vi "Get Boolean.vi"(1 "Name":string) -> (0 "Value":bool)   [LabVIEW 2013]
doc: "Used to retrieve boolean values for use in \"until\" subcommands."
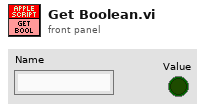
[diagram p1: front panel]
types:
  T1 = enum16{"Wait", "Clear", "Release", "Cock", "Reset"}
  T2 = typedef "WPI_DigitalInputDevRef.ctl" = cluster{"DevStatus":errorcluster, "DIO Channel":T3, "Digital Module":T4}
  T3 = typedef "FPGA_DIOChannel.ctl" = enum8{"DIO 1", "DIO 2", "DIO 3", "DIO 4", "DIO 5", "DIO 6", "DIO 7", "DIO 8", "DIO 9", "DIO 10", "DIO 11", "DIO 12", "DIO 13", "DIO 14", "Invalid"}
  T4 = typedef "FPGA_TypedefDigitalModule.ctl" = enum16{"Digital Module 1", "Digital Module 2"}
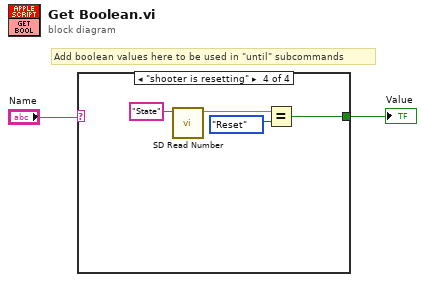
[diagram p0: block diagram]
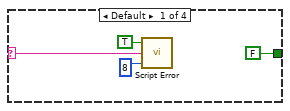
[diagram p2: hidden frame]
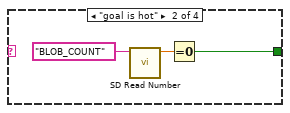
[diagram p3: hidden frame]
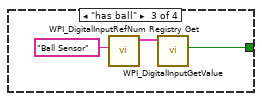
[diagram p4: hidden frame]
diagram:
  # "Add boolean values here to be used in \"until\" subcommands"
  n1 = case shown="\"shooter is resetting\"" "Name" {
    selector: "Name" -> [w3 _ _ _]
    tunnel: [FALSE w7 w10 w13] -> w2
    frame Default {
      n2 = call "Script Error.vi"("Error?"=TRUE, "Error Details"=w3, "Error Code"=8) -> ()  [unwired: 3 in]
    }
    frame "goal is hot" {
      n3 = call <vilib>:"SD Read Number.vi"("Name"="BLOB_COUNT") -> ("Numeric"=w8:dbl)  [unwired: 8 in, 2 out]
      n4 = Equal To 0?(x=w8) -> (x = 0?=w7:bool)
    }
    frame "has ball" {
      n5 = call <vilib>:"WPI_DigitalInputRefNum Registry Get.vi"("refnum name"="Ball Sensor") -> ("DigitalInputDevRef"=w12:T2)  [unwired: 9 in, 1 out]
      n6 = call <vilib>:"WPI_DigitalInputGetValue.vi"("DigitalInputDevRef"=w12) -> ("Value"=w10:bool)  [unwired: 8 in, 2 out]
    }
    frame "shooter is resetting" {
      n7 = call <vilib>:"SD Read Number.vi"("Name"="State") -> ("Numeric"=w15:dbl)  [unwired: 8 in, 2 out]
      n8 = Equal?(x=w15, y=T1."Reset") -> (x = y?=w13:bool)
    }
  }
  "Value" <- w2
